vi "主程序.vi"() -> ()   [LabVIEW 2023]
panel:
  out "用时（秒）":dbl
  in  "bmp路径":path
  out "剩余旗子":u16
  out "剩余方块":u16
  out "游戏结果":bool
  in  "雷数":u16=20
  out "地图":dbl[][](array[numeric])
  out "雷区":dbl[][](array[numeric])
  out "start":bool
  in  "列":u16=10
  in  "行":u16=10
  out "图片":picture
  # "目前配置：\n1608*872\n最大50列，27行"
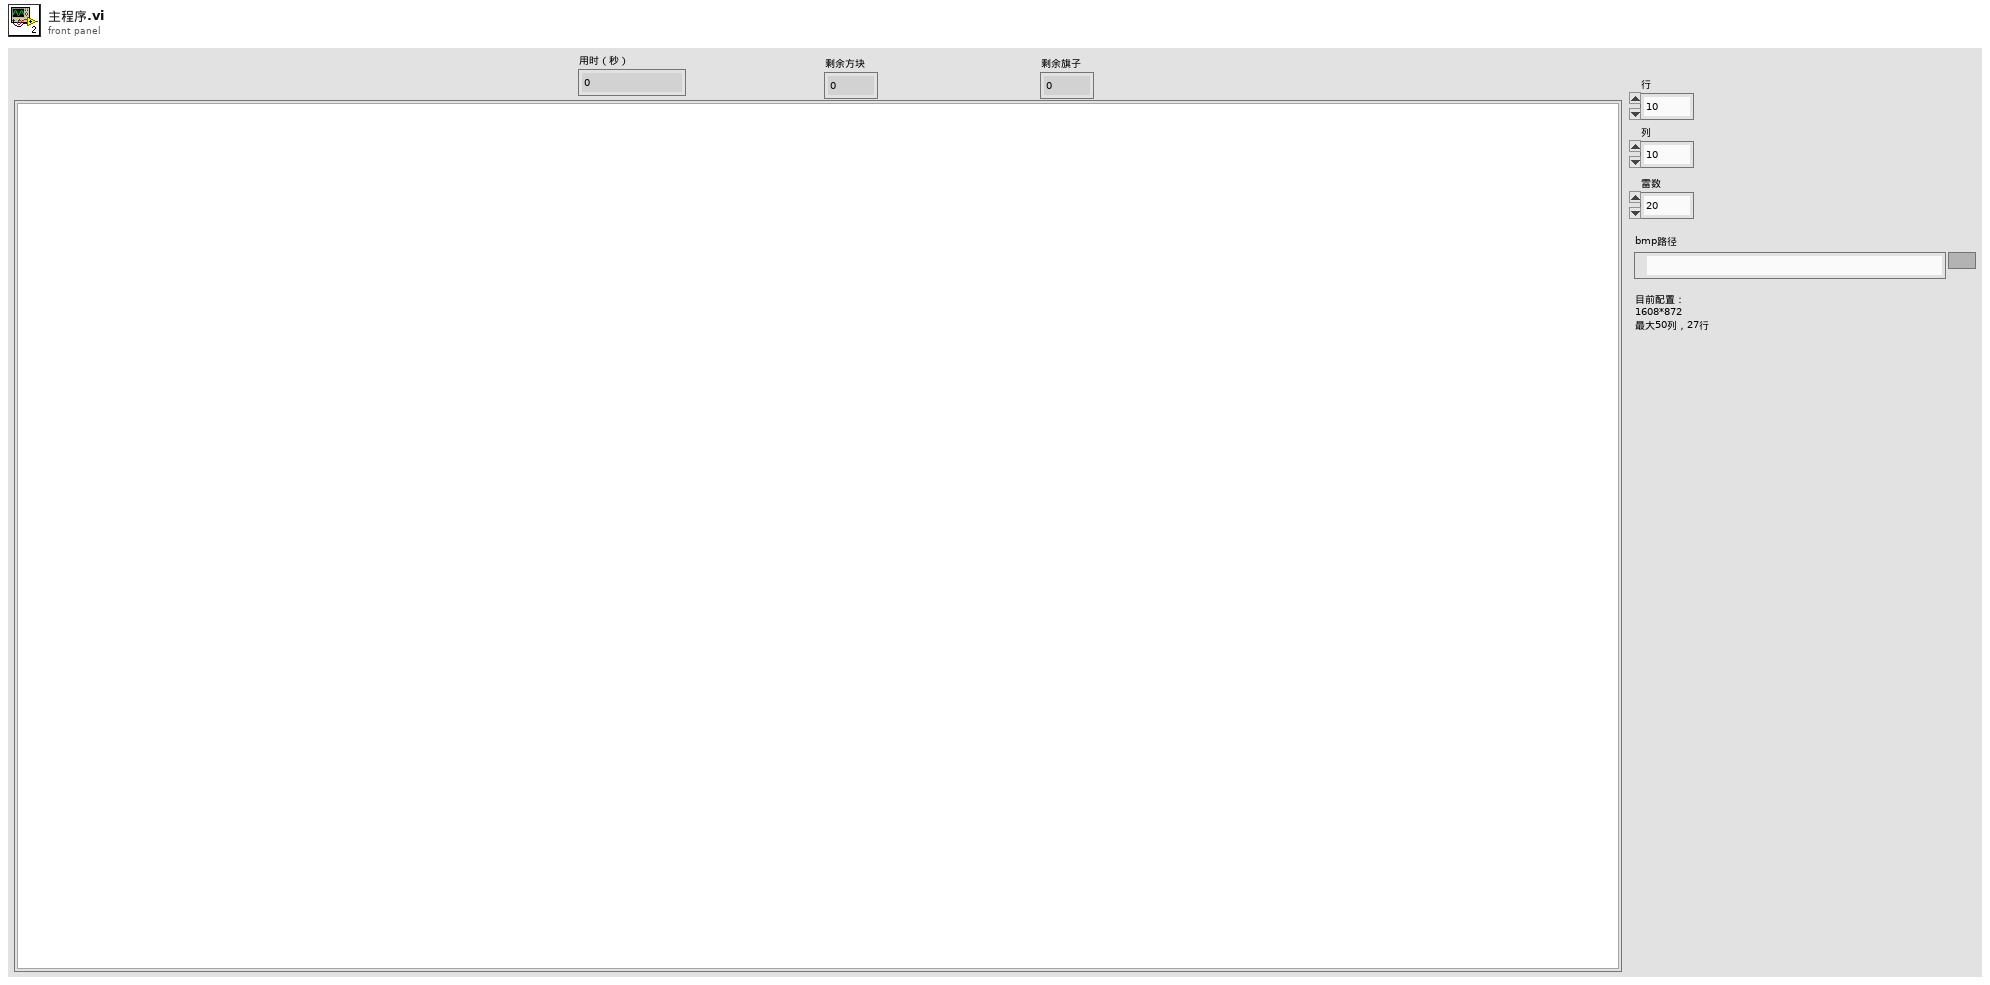
[diagram p1: front panel]
types:
  T1 = cluster{"数组":i32[][][], "colors":u32[], "mask":u8[]}
  T2 = typedef "LVPoint32TypeDef.ctl" = cluster{"Horizontal":i32, "Vertical":i32}
  T3 = typedef "LVPositionTypeDef.ctl" = cluster{"Left":i32, "Top":i32}
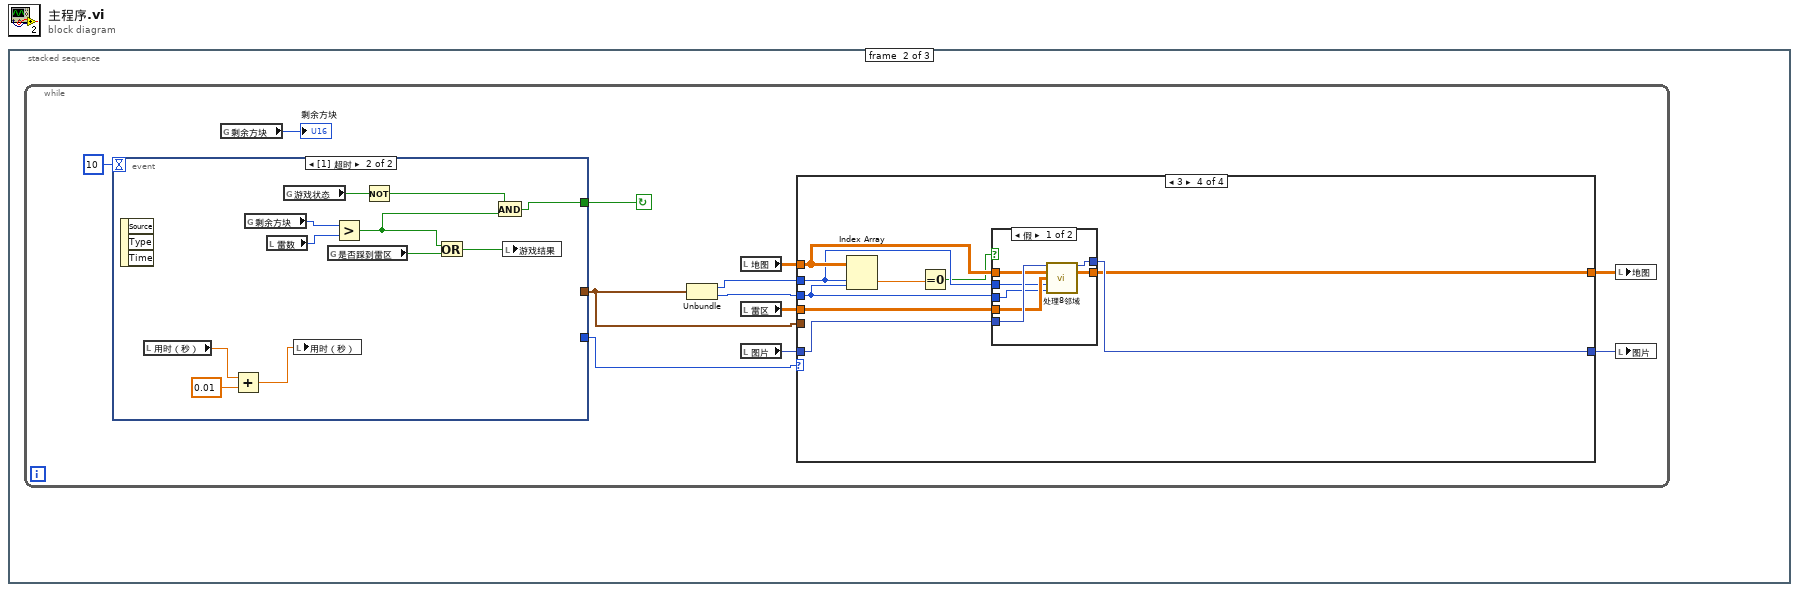
[diagram p0: block diagram]
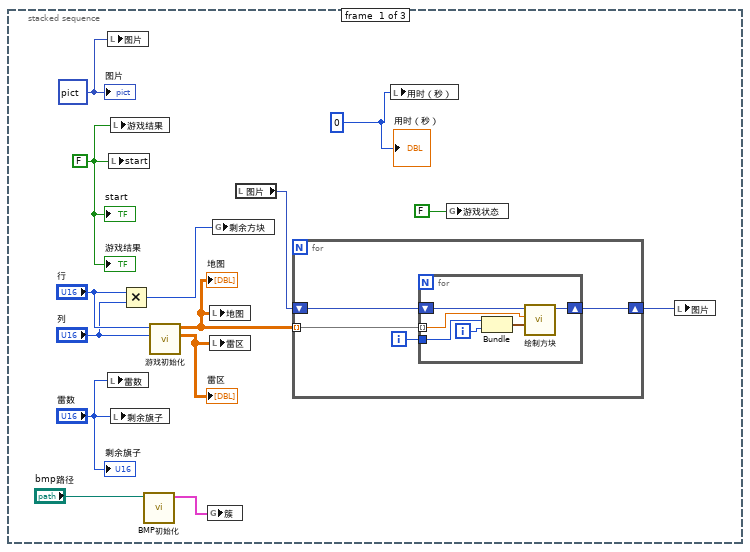
[diagram p2: hidden frame]
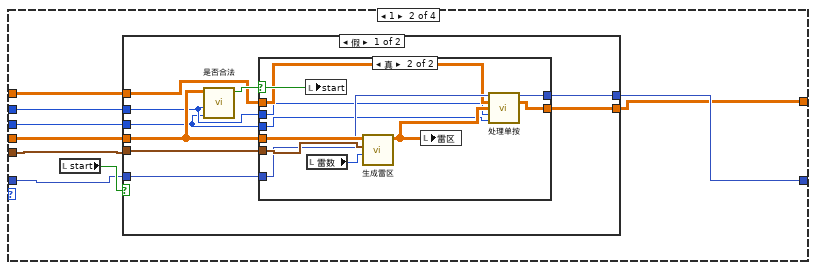
[diagram p4: hidden frame]
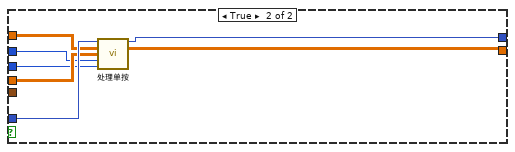
[diagram p6: hidden frame]
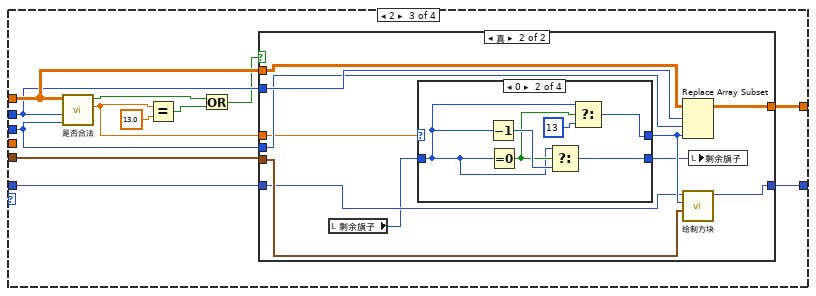
[diagram p7: hidden frame]
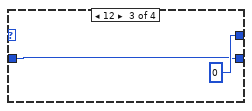
[diagram p10: hidden frame]
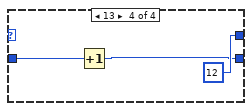
[diagram p11: hidden frame]
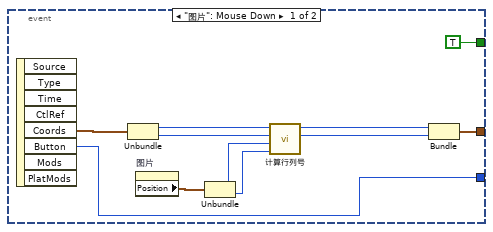
[diagram p13: hidden frame]
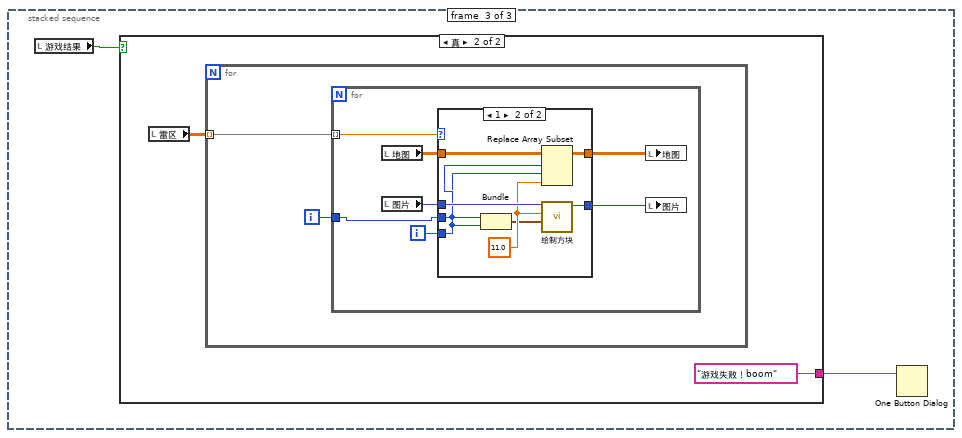
[diagram p14: hidden frame]
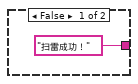
[diagram p15: hidden frame]
diagram:
  n1 = stacked-sequence {
    frame #0 {
      w1 = 0
      w7 = FALSE
      w5 = picture data[5B] ("原图片")
      n2 = local write "图片"(w5) -> ()
      n3 = local write "雷数"("雷数") -> ()
      n4 = local write "start"(w7) -> ()
      n5 = local write "游戏结果"(w7) -> ()
      n6 = local write "剩余旗子"("雷数") -> ()
      n7 = Multiply(x="行", y="列") -> (x*y=w8:u16)
      n8 = call "BMP初始化.vi"("path to BMP file"="bmp路径") -> ("簇"=w10:T1)  [unwired: 10 in]
      n9 = call "游戏初始化.vi"("列数"="列", "行数"="行") -> ("雷区"=w14:dbl[][], "地图"=w13:dbl[][])  [unwired: 8 in]
      "雷区" <- w14
      "地图" <- w13
      n10 = global write "全局变量.vi" "簇"(w10) -> ()
      n11 = local write "地图"(w13) -> ()
      n12 = local write "雷区"(w14) -> ()
      n13 = global write "全局变量.vi" "剩余方块"(w8) -> ()
      n14 = local read "图片"() -> (w12:picture)
      n15 = for {
        tunnel: w13 -> [w18] mode=indexing
        shift-right: [w15] -> w11
        shift-left: w12 -> [w16]
        i -> [w17]
        n16 = for {
          tunnel: w18 -> [w22] mode=indexing
          tunnel: w17 -> [w23]
          shift-right: [w19] -> w15
          shift-left: w16 -> [w20]
          i -> [w24]
          n17 = Bundle(w23, w24) -> (w21:cluster{i32, i32})  [unwired: 1 in]
          n18 = call "绘制方块.vi"("簇"=w21, "ID"=w22, "picture"=w20) -> ("new picture"=w19:picture)  [unwired: 8 in]
        }
      }
      n19 = local write "用时（秒）"(w1) -> ()
      n20 = global write "全局变量.vi" "游戏状态"(FALSE ("游戏状态")) -> ()
      n21 = local write "图片"(w11) -> ()
      "start" <- w7
      "图片" <- w5
      "游戏结果" <- w7
      "剩余旗子" <- "雷数"
      "用时（秒）" <- w1
    }
    frame #1 {
      n22 = while {
        stop <- w34 continue-if-true
        n23 = event shown="[1] 超时" {
          selector: _ -> [_ _]
          dyn-events: _ -> [_ _]
          timeout: 10 -> [_ _]
          tunnel: [w142 _] -> w36
          tunnel: [w139 _] -> w35
          tunnel: [TRUE w147] -> w34
          event "图片": Mouse Down {
            n24 = event-data() -> ("Coords"=w143:T2, "Button"=w142:u16)  [unwired: 1 in, 6 out]
            n25 = Unbundle(w143) -> ("Horizontal"=w138:i32, "Vertical"=w137:i32)
            n26 = property on="图片" class="Pict"() -> ("Position"=w136:T3)  [unwired: 2 in, 2 out]
            n27 = Unbundle(w136) -> ("Left"=w135:i32, "Top"=w134:i32)
            n28 = call "计算行列号.vi"("垂直偏移"=w134, "水平偏移"=w135, "垂直"=w137, "水平"=w138) -> ("列"=w140:i16, "行"=w141:i16)  [unwired: 6 in]
            n29 = Bundle("行"=w141, "列"=w140) -> (w139:cluster{"行":i16, "列":i16})  [unwired: 1 in]
          }
          event Timeout {
            n30 = event-data() -> ()  [unwired: 1 in, 3 out]
            n31 = local read "用时（秒）"() -> (w153:dbl)
            n32 = Add(x=w153, y=0.01) -> (x+y=w152:dbl)
            n33 = global read "全局变量.vi" "剩余方块"() -> (w151:u16)
            n34 = local read "雷数"() -> (w150:u16)
            n35 = global read "全局变量.vi" "游戏状态"() -> (w149:bool)
            n36 = local write "用时（秒）"(w152) -> ()
            n37 = global read "全局变量.vi" "是否踩到雷区"() -> (w146:bool)
            n38 = Greater?(x=w151, y=w150) -> (0:w145:bool)
            n39 = Not(x=w149) -> (.not. x?=w148:bool)
            n40 = Or(x=w145, y=w146) -> (x .or. y?=w144:bool)
            n41 = And(x=w148, y=w145) -> (x .and. y?=w147:bool)
            n42 = local write "游戏结果"(w144) -> ()
          }
        }
        n43 = global read "全局变量.vi" "剩余方块"() -> (→"剩余方块":u16)
        n44 = Unbundle(w35) -> ("行"=w27:i16, "列"=w26:i16)
        n45 = local read "地图"() -> (w32:dbl[][])
        n46 = local read "雷区"() -> (w31:dbl[][])
        n47 = local read "图片"() -> (w29:picture)
        n48 = case shown="3" w36 {
          tunnel: w32 -> [w38 w41 w84 w119]
          tunnel: w31 -> [_ w46 _ w122]
          tunnel: w35 -> [_ w45 w87 _]
          tunnel: [w38 w39 w88 w120] -> w30
          tunnel: w29 -> [w37 w42 w85 w123]
          tunnel: [w37 w40 w86 w121] -> w28
          tunnel: w27 -> [_ w44 w83 w118]
          tunnel: w26 -> [_ w43 w82 w117]
          frame 0, Default {
          }
          frame 1 {
            n49 = local read "start"() -> (w47:bool)
            n50 = case shown="假" w47 {
              tunnel: w45 -> [w56 _]
              tunnel: w46 -> [w55 w74]
              tunnel: w44 -> [w51 w73]
              tunnel: w43 -> [w50 w72]
              tunnel: w42 -> [w53 w76]
              tunnel: w41 -> [w52 w75]
              tunnel: [w49 w71] -> w40
              tunnel: [w48 w70] -> w39
              frame False {
                n51 = call "是否合法.vi"("列"=w50, "行"=w51, "地图"=w55) -> ("是否合法"=w54:bool)  [unwired: 7 in, 1 out]
                n52 = case shown="真" w54 {
                  selector: w54 -> [_ w66]
                  tunnel: w56 -> [_ w69]
                  tunnel: w55 -> [_ w67]
                  tunnel: w53 -> [w58 w65]
                  tunnel: w52 -> [w57 w64]
                  tunnel: w51 -> [_ w62]
                  tunnel: w50 -> [_ w61]
                  tunnel: [w58 w60] -> w49
                  tunnel: [w57 w59] -> w48
                  frame False {
                  }
                  frame True {
                    n53 = local write "start"(w66) -> ()
                    n54 = local read "雷数"() -> (w68:u16)
                    n55 = call "生成雷区.vi"("雷数"=w68, "firstPT"=w69, "输入"=w67) -> ("输出"=w63:dbl[][])  [unwired: 8 in]
                    n56 = local write "雷区"(w63) -> ()
                    n57 = call "处理单按.vi"("图片"=w65, "地图"=w64, "雷区"=w63, "行"=w62, "列"=w61) -> ("图片 2"=w60:picture, "地图 2"=w59:dbl[][])  [unwired: 7 in, 2 out]
                  }
                }
              }
              frame True {
                n58 = call "处理单按.vi"("图片"=w76, "地图"=w75, "雷区"=w74, "行"=w73, "列"=w72) -> ("图片 2"=w71:picture, "地图 2"=w70:dbl[][])  [unwired: 7 in, 2 out]
              }
            }
          }
          frame 2 {
            n59 = call "是否合法.vi"("列"=w82, "行"=w83, "地图"=w84) -> ("元素"=w77:dbl, "是否合法"=w79:bool)  [unwired: 7 in]
            n60 = Equal?(x=w77, y=13.0) -> (x = y?=w80:bool)
            n61 = Or(x=w79, y=w80) -> (x .or. y?=w78:bool)
            n62 = case shown="真" w78 {
              tunnel: [w89 w101] -> w88
              tunnel: w87 -> [_ w100]
              tunnel: [w90 w98] -> w86
              tunnel: w85 -> [w90 w97]
              tunnel: w84 -> [w89 w94]
              tunnel: w83 -> [_ w93]
              tunnel: w82 -> [_ w92]
              tunnel: w77 -> [_ w91]
              frame False {
              }
              frame True {
                n63 = local read "剩余旗子"() -> (w96:u16)
                n64 = case shown="0" w91 {
                  selector: w91 -> [w103 _ _ _]
                  tunnel: [w103 w104 0 12] -> w99
                  tunnel: w96 -> [w102 w105 w110 w113]
                  tunnel: [w102 w108 w110 w112] -> w95
                  frame -1, Default {
                  }
                  frame 0 {
                    n65 = Decrement(x=w105) -> (x-1=w109:u16)
                    n66 = Equal To 0?(x=w105) -> (x = 0?=w106:bool)
                    n67 = Select(t=w105, s=w106, f=w109) -> (s? t:f=w108:u16)
                    n68 = Select(t=w105, s=w106, f=13) -> (s? t:f=w104:i32)
                  }
                  frame 12 {
                  }
                  frame 13 {
                    n69 = Increment(x=w113) -> (x+1=w112:u16)
                  }
                }
                n70 = Replace Array Subset(array=w94, new element=w99, index (row)=w93, index (col)=w92) -> (w101:dbl[][])
                n71 = call "绘制方块.vi"("簇"=w100, "ID"=w99, "picture"=w97) -> ("new picture"=w98:picture)  [unwired: 8 in]
                n72 = local write "剩余旗子"(w95) -> ()
              }
            }
          }
          frame 3 {
            n73 = Index Array(array=w119, index (row)=w118, index (col)=w117) -> (element=w116:dbl)
            n74 = Equal To 0?(x=w116) -> (x = 0?=w115:bool)
            n75 = case shown="假" w115 {
              tunnel: w123 -> [w130 w132]
              tunnel: w122 -> [w129 _]
              tunnel: [w128 w132] -> w121
              tunnel: [w127 w131] -> w120
              tunnel: w119 -> [w126 w131]
              tunnel: w118 -> [w125 _]
              tunnel: w117 -> [w124 _]
              frame False {
                n76 = call "处理8邻域.vi"("图片"=w130, "地图"=w126, "雷区"=w129, "行"=w125, "列"=w124) -> ("图片 2"=w128:picture, "地图 2"=w127:dbl[][])  [unwired: 9 in]
              }
              frame True {
              }
            }
          }
        }
        n77 = local write "地图"(w30) -> ()
        n78 = local write "图片"(w28) -> ()
      }
    }
    frame #2 {
      n79 = local read "游戏结果"() -> (w156:bool)
      n80 = case shown="真" w156 {
        tunnel: ["扫雷成功！" "游戏失败！boom"] -> w155
        frame False {
        }
        frame True {
          n81 = local read "雷区"() -> (w159:dbl[][])
          n82 = for {
            tunnel: w159 -> [w161] mode=indexing
            i -> [w160]
            n83 = for {
              tunnel: w161 -> [w168] mode=indexing
              tunnel: w160 -> [w166]
              i -> [w167]
              n84 = local read "地图"() -> (w162:dbl[][])
              n85 = local read "图片"() -> (w164:picture)
              n86 = case shown="1" w168 {
                tunnel: w167 -> [_ w172]
                tunnel: w166 -> [_ w173]
                tunnel: [w170 w175] -> w165
                tunnel: w164 -> [w170 w176]
                tunnel: [w169 w177] -> w163
                tunnel: w162 -> [w169 w178]
                frame 0, Default {
                }
                frame 1 {
                  w174 = 11.0 ("新元素/子数组")
                  n87 = Bundle(w173, w172) -> (w171:cluster{i32, i32})  [unwired: 1 in]
                  n88 = Replace Array Subset(array=w178, new element=w174, index (row)=w173, index (col)=w172) -> (w177:dbl[][])
                  n89 = call "绘制方块.vi"("簇"=w171, "ID"=w174, "picture"=w176) -> ("new picture"=w175:picture)  [unwired: 8 in]
                }
              }
              n90 = local write "地图"(w163) -> ()
              n91 = local write "图片"(w165) -> ()
            }
          }
        }
      }
      n92 = One Button Dialog(message=w155) -> ()  [unwired: 1 in, 1 out]
    }
  }
